vi "request recovery.vi"(8 "error in":errorcluster, 10 "recovery request":T1={"module ref"=refnum, "engine reference"=0, "original run flags"=0, "attempts allowed"=1, "cfg ref"=refnum}, 11 "async exec ref in":T2) -> (0 "error out":errorcluster, 3 "async exec ref out":T2)   [LabVIEW 2013]
uses:
  Runtime/async command notification.ctl
  async executor.lvlib
  <vilib>/NI/Tag Bus/table/data table.ctl
  <vilib>/NI/Tag Bus/table/data table.lvlib
  <vilib>/NI/Tag Bus/buffer exchange/buffer reference.ctl
  <vilib>/NI/Tag Bus/buffer exchange/tag bus buffer exchange.lvlib
  <vilib>/NI/Tag Bus Module Framework/runtime/error classification.ctl
  <vilib>/NI/Tag Bus Module Framework/runtime/TBM module execution interface.lvclass
  Runtime/async error info.ctl
  asynchronous executor reference.ctl
  <vilib>/NI/Tag Bus Module Framework/module configuration/TBM module configuration.lvclass
  worker library/recovery request.ctl
  worker library/worker pool.lvlib
  message to executor.ctl
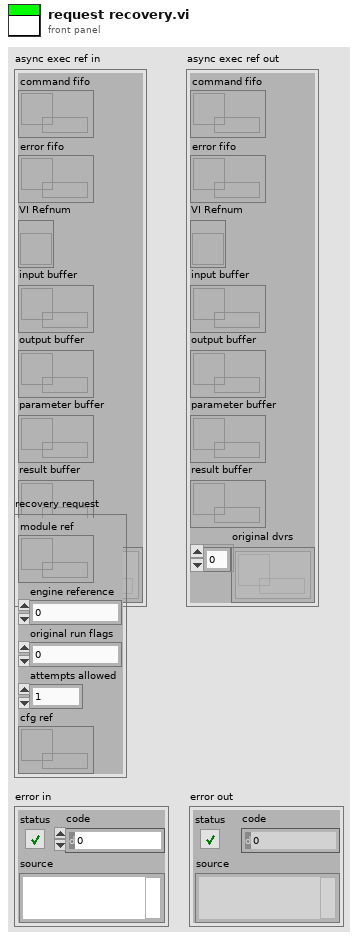
[diagram p1: front panel]
types:
  T1 = typedef "worker pool.lvlib/recovery request.ctl" = cluster{"module ref":refnum<data-value>, "engine reference":i32, "original run flags":u8, "attempts allowed":u16, "cfg ref":refnum<data-value>}
  T2 = typedef "async executor.lvlib/asynchronous executor reference.ctl" = cluster{"command fifo":refnum<k33>, "error fifo":refnum<k33>, "VI Refnum":refnum<vi>, "input buffer":refnum<k33>, "output buffer":refnum<k33>, "parameter buffer":refnum<k33>, "result buffer":refnum<k33>, "original dvrs":T3[]}
  T3 = typedef "tag bus buffer exchange.lvlib/buffer reference.ctl" = refnum<data-value>
  T4 = typedef "async executor.lvlib/async command notification.ctl" = enum16{"stop", "input", "process", "output"}
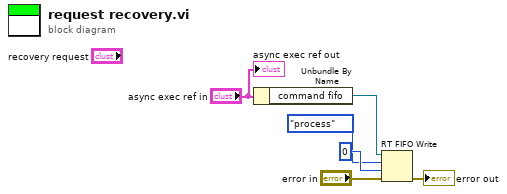
[diagram p0: block diagram]
diagram:
  n1 = Unbundle By Name("async exec ref in") -> ("command fifo"=w3:refnum<k33>)
  n2 = RT FIFO Write(0:w3, 1:async_command_notification."process" ("element"), 2:0 ("timeout in ms (0)"), 3:"error in") -> (11:→"error out":errorcluster)  [unwired: 1 in, 3 out]
  "async exec ref out" <- "async exec ref in"
